vi "Create Counter Driven Output Module.vi"   [LabVIEW 2020, in "Scan Engine Scripting.lvlib"]
doc: "Creates and configures an instance of a counter driven output module that can be used to set a slot in a Scan Engine custom device chassis."
uses:
  Scan Engine Scripting.lvlib
  Modules/NI 9474/NI 9474.lvclass
  Modules/NI 9475/NI 9475.lvclass
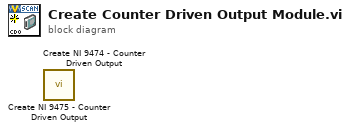
[diagram p0: block diagram]
diagram:
  n1 = call "Create NI 9475 - Counter Driven Output.vi"() -> ()  [unwired: 10 in, 2 out]
  n2 = call "Create NI 9474 - Counter Driven Output.vi"() -> ()  [unwired: 10 in, 2 out]
